vi "Pre Launch Init.vi"(11 "ImageHandler in":refnum<class "ImageHandler.lvclass">) -> (0 "error out":errorcluster, 3 "ImageHandler out":refnum<class "ImageHandler.lvclass">)   [LabVIEW 2022 SP3, in "ImageHandler.lvlib" / "ImageHandler.lvclass"]
doc: "(<B>Filename</B>: Actor Framework.lvlib:Actor.lvclass:Pre Launch Init.vi)\n\nDefines behavior that occurs after the Launch Actor method is invoked but before the actor's Actor Core method begins running.\n\nThe Pre Launch Init method is guaranteed to finish before the Launch Actor method returns to its caller and before the actor itself receives any messages. Any references that the Pre Launch Init method obtains are guaranteed to have the same lifetime as the actor itself. Any errors that the Pre Launch Init method returns will abort the launch.\n\nBy default, this method does nothing. A descendant class may override it to define behavior."
uses:
  ImageHandler.lvclass
  ImageHandler.lvclass/ImageHandler.ctl
  <vilib>/ActorFramework/Actor/Actor.lvclass
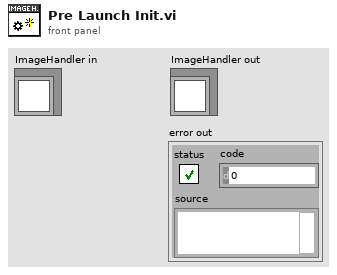
[diagram p1: front panel]
types:
  T1 = typedef "Image Type" = u32
  T2 = typedef "IMAQ Image.ctl" = refnum<image>
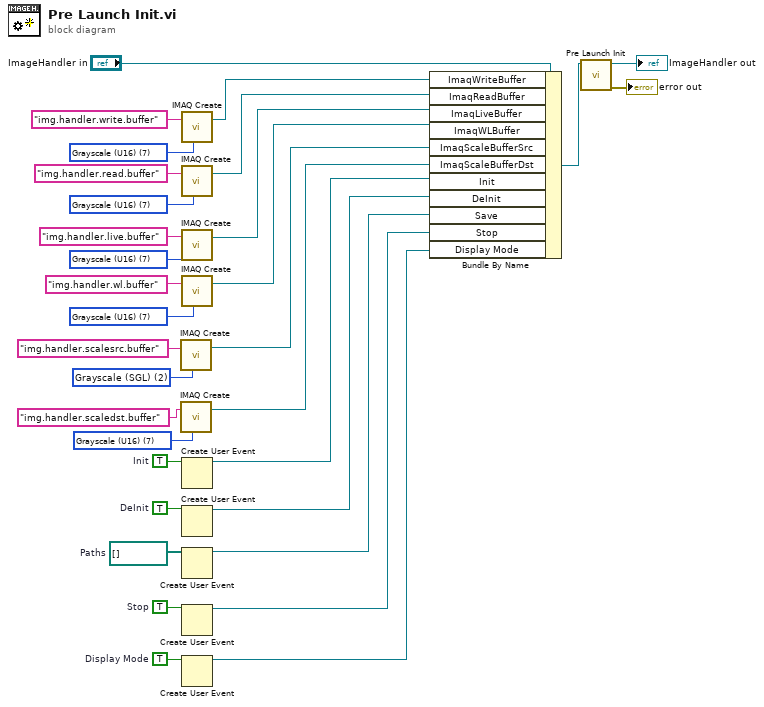
[diagram p0: block diagram]
diagram:
  w5 = T1 7 items=["Grayscale (U8)", "Grayscale (I16)", "Grayscale (SGL)", "Complex (CSG)", "RGB (U32)", "HSL (U32)", "RGB (U64)", "Grayscale (U16)"] ("Image Type")
  w6 = T1 2 items=["Grayscale (U8)", "Grayscale (I16)", "Grayscale (SGL)", "Complex (CSG)", "RGB (U32)", "HSL (U32)", "RGB (U64)", "Grayscale (U16)"] ("Image Type")
  w9 = T1 7 items=["Grayscale (U8)", "Grayscale (I16)", "Grayscale (SGL)", "Complex (CSG)", "RGB (U32)", "HSL (U32)", "RGB (U64)", "Grayscale (U16)"] ("Image Type")
  w11 = TRUE  # Display Mode
  w13 = T1 7 items=["Grayscale (U8)", "Grayscale (I16)", "Grayscale (SGL)", "Complex (CSG)", "RGB (U32)", "HSL (U32)", "RGB (U64)", "Grayscale (U16)"] ("Image Type")
  w19 = TRUE  # Stop
  w20 = path[] []  # Paths
  w21 = TRUE  # DeInit
  w22 = TRUE  # Init
  w25 = T1 7 items=["Grayscale (U8)", "Grayscale (I16)", "Grayscale (SGL)", "Complex (CSG)", "RGB (U32)", "HSL (U32)", "RGB (U64)", "Grayscale (U16)"] ("Image Type")
  w26 = T1 7 items=["Grayscale (U8)", "Grayscale (I16)", "Grayscale (SGL)", "Complex (CSG)", "RGB (U32)", "HSL (U32)", "RGB (U64)", "Grayscale (U16)"] ("Image Type")
  n1 = call "IMAQ Create"("Image Name"="img.handler.scalesrc.buffer", "Image Type"=w6) -> ("New Image"=w2:T2)  [unwired: 3 in, 1 out]
  n2 = call "IMAQ Create"("Image Name"="img.handler.scaledst.buffer", "Image Type"=w5) -> ("New Image"=w1:T2)  [unwired: 3 in, 1 out]
  n3 = call "IMAQ Create"("Image Name"="img.handler.write.buffer", "Image Type"=w26) -> ("New Image"=w23:T2)  [unwired: 3 in, 1 out]
  n4 = call "IMAQ Create"("Image Name"="img.handler.read.buffer", "Image Type"=w25) -> ("New Image"=w24:T2)  [unwired: 3 in, 1 out]
  n5 = call "IMAQ Create"("Image Name"="img.handler.live.buffer", "Image Type"=w13) -> ("New Image"=w12:T2)  [unwired: 3 in, 1 out]
  n6 = call "IMAQ Create"("Image Name"="img.handler.wl.buffer", "Image Type"=w9) -> ("New Image"=w7:T2)  [unwired: 3 in, 1 out]
  n7 = Create User Event(user event datatype=w22) -> (user event=w18:refnum<user-event>)  [unwired: 1 in, 1 out]
  n8 = Create User Event(user event datatype=w21) -> (user event=w17:refnum<user-event>)  [unwired: 1 in, 1 out]
  n9 = Create User Event(user event datatype=w20) -> (user event=w16:refnum<user-event>)  [unwired: 1 in, 1 out]
  n10 = Create User Event(user event datatype=w19) -> (user event=w15:refnum<user-event>)  [unwired: 1 in, 1 out]
  n11 = Create User Event(user event datatype=w11) -> (user event=w10:refnum<user-event>)  [unwired: 1 in, 1 out]
  n12 = Bundle By Name(cluster="ImageHandler in", "ImaqWriteBuffer"=w23, "ImaqReadBuffer"=w24, "ImaqLiveBuffer"=w12, "ImaqWLBuffer"=w7, "ImaqScaleBufferSrc"=w2, "ImaqScaleBufferDst"=w1, "Init"=w18, "DeInit"=w17, "Save"=w16, "Stop"=w15, "Display Mode"=w10) -> (w29:refnum<class "ImageHandler.lvclass">)
  n13 = call-parent "Pre Launch Init.vi"("Actor in"=w29) -> ("error out"=→"error out":errorcluster, "Actor out"=→"ImageHandler out":refnum<class "ImageHandler.lvclass">)  [unwired: 9 in]
